vi "G#SubClass1_Create.vi"(0 "reference in":refnum<class "G#SubClass1.lvclass">, 1 "object name":string, 4 "no registration":bool, 5 "error in (no error)":errorcluster, 6 "create method":T1=enum."Create or look up existing", 7 "user counter":bool=TRUE) -> (12 "created new?":bool, 14 "reference out":refnum<class "G#SubClass1.lvclass">, 19 "error out":errorcluster)   [LabVIEW 2020, in "G#SubClass1.lvclass"]
doc: "Constructor."
uses:
  G#SubClass1.lvclass
  C:/Program Files (x86)/National Instruments/LabVIEW 2020/vi.lib/addons/_AddQ/G#Object/G#Object.lvclass
  C:/Projects/GsharpGIT/Verification/TestCases/TestClasses/G#BaseClass1_class/G#BaseClass1.lvclass
  <vilib>/addons/_AddQ/G#Object/utils/G#Object_CreateMethod.ctl
  <vilib>/addons/_AddQ/G#Object/G#Object.lvclass
  G#BaseClass1_class/G#BaseClass1.lvclass
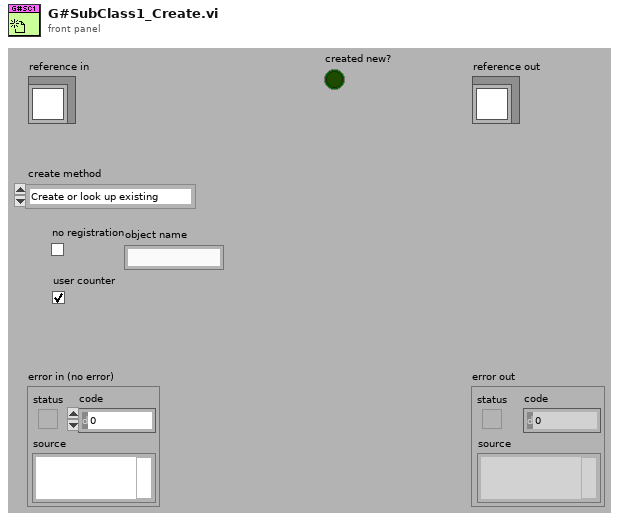
[diagram p1: front panel]
types:
  T1 = typedef "G#Object.lvclass/G#Object_CreateMethod.ctl" = enum16{"Create", "Create or look up existing", "Look up existing"}
  T2 = typedef "G#SubClass1.lvclass/ObjectAttributesRef.ctl" = refnum<data-value>
  T3 = typedef "G#SubClass1.lvclass/ObjectAttributes.ctl" = cluster{"SubNumeric":dbl, "TestQueue":refnum<queue>}
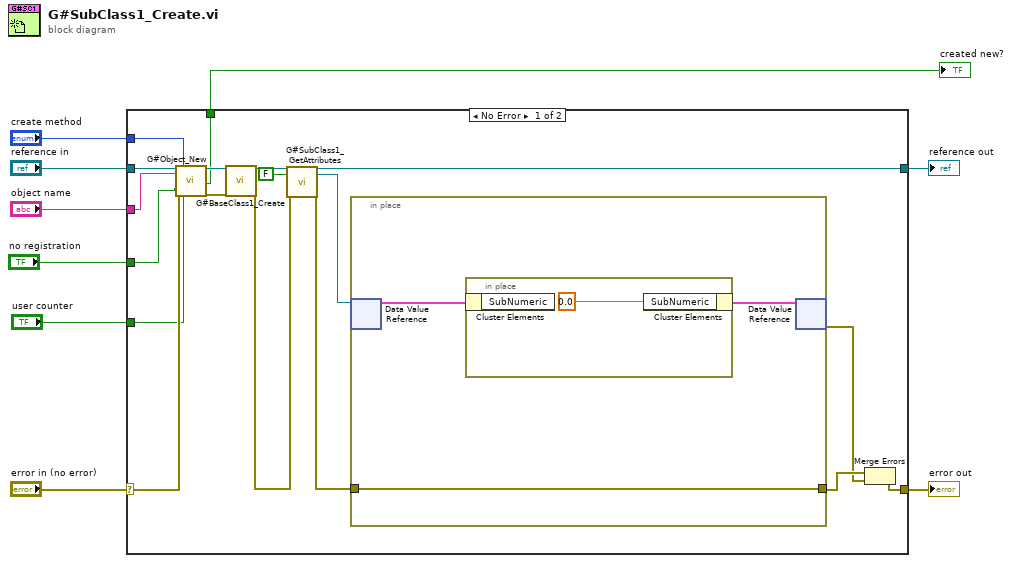
[diagram p0: block diagram]
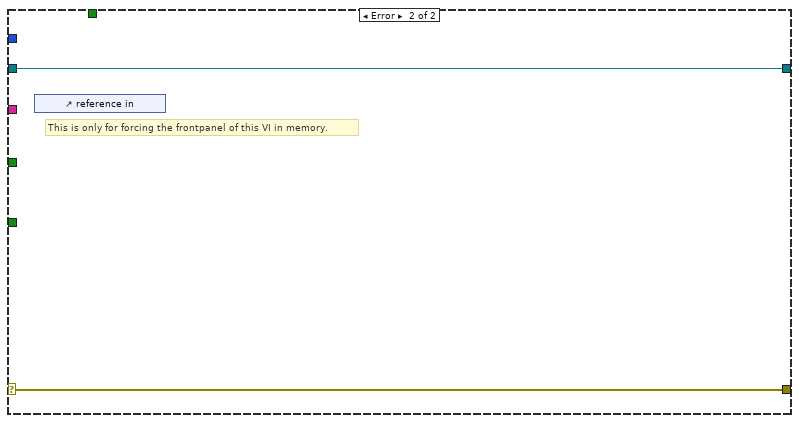
[diagram p2: hidden frame]
diagram:
  n1 = case shown="No Error" "error in (no error)" {
    selector: "error in (no error)" -> [w26 w33]
    tunnel: [w25 w33] -> w8
    tunnel: [w14 w32] -> w6
    tunnel: "reference in" -> [w27 w32]
    tunnel: "create method" -> [w20 _]
    tunnel: "object name" -> [w19 _]
    tunnel: "no registration" -> [w18 _]
    tunnel: "user counter" -> [w17 _]
    tunnel: [w16 _] -> w1
    frame No Error {
      n2 = call <vilib>:"G#Object_New.vi"("reference in"=w27, "object name"=w19, "no registration? (F)"=w18, "error in (no error)"=w26, "create method"=w20, "user counter (T)?"=w17) -> ("reference out"=w24:refnum<class "G#SubClass1.lvclass">, "created new?"=w16:bool, "error out"=w23:errorcluster)  [unwired: 11 in]
      n3 = call "G#BaseClass1_Create.vi"("reference in"=w24, "error in (no error)"=w23) -> ("reference out"=w15:refnum<class "G#SubClass1.lvclass">, "error out"=w12:errorcluster)  [unwired: 15 in, 1 out]
      n4 = call "G#SubClass1_GetAttributes.vi"("reference in"=w15, "return data? (T)"=FALSE, "error in (no error)"=w12) -> ("reference out"=w14:refnum<class "G#SubClass1.lvclass">, "attributes ref"=w10:T2, "error out"=w11:errorcluster)  [unwired: 13 in, 1 out]
      n5 = in-place {
        in-place-border: w11 -> [w28]
        in-place-border: [w28] -> w22
        n6 = in-place-dvr #1(w10) -> (w29:T3)  [unwired: 1 out]
        n7 = in-place {
          n8 = in-place-cluster #2(w29) -> ()  [unwired: 1 out]
          n9 = in-place-cluster #2("SubNumeric"=0.0 ("Numeric")) -> (w30:T3)
        }
        n10 = in-place-dvr #1(w30) -> (w21:errorcluster)  [unwired: 1 out]
      }
      n11 = Merge Errors(w22, w21) -> (w25:errorcluster)
    }
    frame Error {
      # "This is only for forcing the frontpanel of this VI in memory."
      n12 = control-ref of="reference in"() -> ()  [unwired: 1 out]
    }
  }
  "error out" <- w8
  "reference out" <- w6
  "created new?" <- w1
